vi "test_using_array_to_csv.vi"() -> ()   [LabVIEW 2013]
panel:
  out "error out":errorcluster
  out "Baseline":i16
  out "Stdev":i16
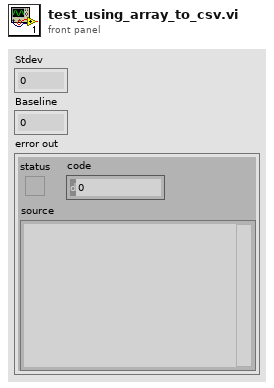
[diagram p1: front panel]
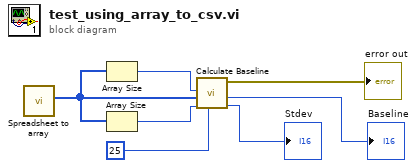
[diagram p0: block diagram]
diagram:
  n1 = call "Spreadsheet to array.vi"() -> ("Array"=w2:u16[])  [unwired: 8 in, 3 out]
  n2 = Array Size(array=w2) -> (size(s)=w1:i32)
  n3 = Array Size(array=w2) -> (size(s)=w7:i32)
  n4 = call "Calculate Baseline.vi"("baselineThreshold"=u16 25, "traceLength"=w7, "data_12_bit"=w2, "baselineLength"=w1) -> ("Stdev"=→"Stdev":i16, "Baseline"=→"Baseline":i16, "error out"=→"error out":errorcluster)  [unwired: 5 in]
